vi "convert from time clust to ns start BAE2.vi"(1 "time cluster":T1={"day [max]"=0, "hour [23]"=0, "min [59]"=0, "sec [59]"=1, "msec [999]"=0, "usec [999]"=0, "nsec [1000]"=0}) -> (8 "time (nsec)":i64=1000)   [LabVIEW 2014]
doc: "This subvi converts a typedefined U32 time cluster in a format of: [weeks, days, hours (24), min, sec, msec, usec, and nsec] to nsec \n\nIt uses a I64 format for the time in nsec and thus is limited to 2^63-1 nsec before rolling over, meaning that it wont reset for years.\n\nPaul K Dixon\nP350\nCSUSB Physics"
uses:
  typedefs/time cluster typedef.ctl
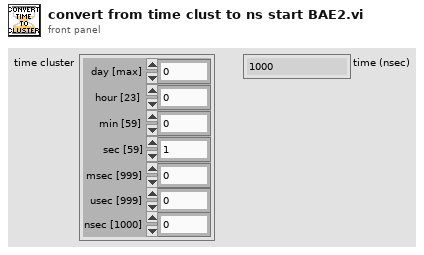
[diagram p1: front panel]
types:
  T1 = typedef "time cluster typedef.ctl" = cluster{"day [max]":u32, "hour [23]":u32, "min [59]":u32, "sec [59]":u32, "msec [999]":u32, "usec [999]":u32, "nsec [1000]":u32}
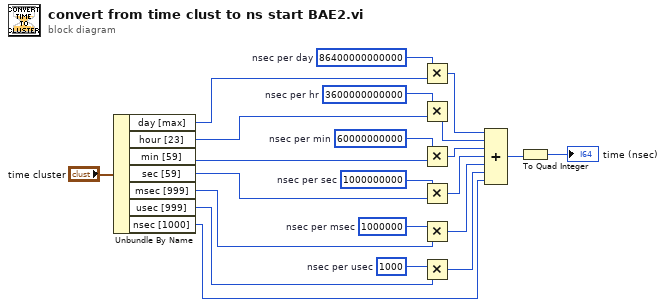
[diagram p0: block diagram]
diagram:
  w16 = i64 1000  # nsec per usec
  w17 = i64 1000000  # nsec per msec
  w18 = i64 1000000000  # nsec per sec
  w19 = i64 60000000000  # nsec per min
  w20 = i64 3600000000000  # nsec per hr
  w21 = i64 86400000000000  # nsec per day
  n1 = Unbundle By Name("time cluster") -> ("day [max]"=w15:u32, "hour [23]"=w14:u32, "min [59]"=w13:u32, "sec [59]"=w12:u32, "msec [999]"=w11:u32, "usec [999]"=w10:u32, "nsec [1000]"=w9:u32)
  n2 = Multiply(x=w21, y=w15) -> (x*y=w8:i64)
  n3 = Multiply(x=w20, y=w14) -> (x*y=w7:i64)
  n4 = Multiply(x=w19, y=w13) -> (x*y=w6:i64)
  n5 = Multiply(x=w18, y=w12) -> (x*y=w5:i64)
  n6 = Multiply(x=w17, y=w11) -> (x*y=w4:i64)
  n7 = Multiply(x=w16, y=w10) -> (x*y=w3:i64)
  n8 = Compound Arithmetic op=ADD(w8, w7, w6, w5, w4, w3, w9) -> (w1:i64)
  n9 = To Quad Integer(1:w1) -> (0:→"time (nsec)":i64)
